vi "Labview Demo 2.vi"() -> ()   [LabVIEW 2016]
uses:
  C:/Program Files (x86)/Doodlebase/Transformer/Schemaport.Doodlebase.Transformer.dll
  Program Files (x86)/Doodlebase/Transformer/Schemaport.Doodlebase.Transformer.dll
panel:
  out "Network Success":bool
  in  "Variables":dbl
  in  "File Path Directory":path
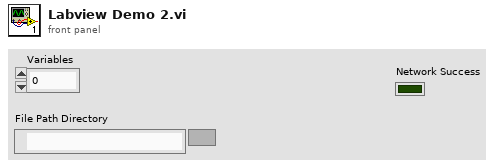
[diagram p1: front panel]
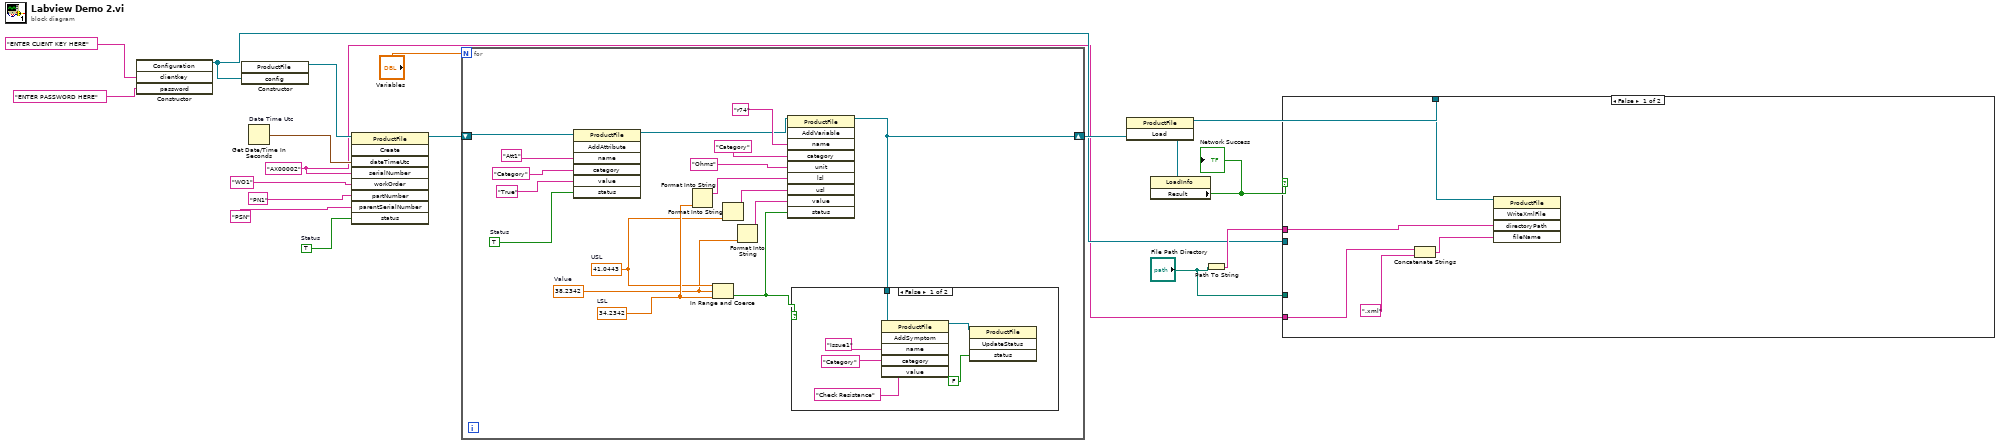
[diagram p0: block diagram]
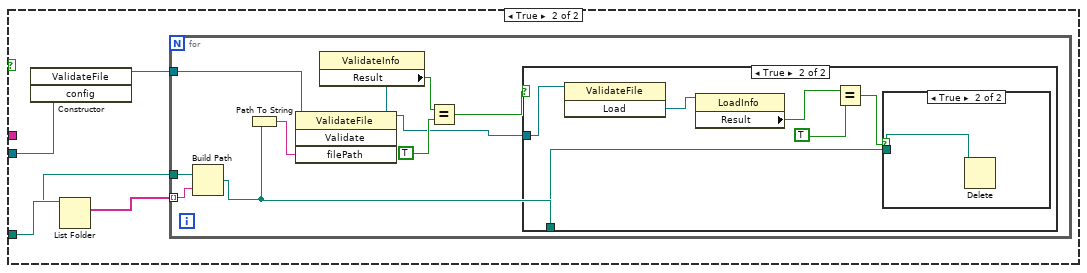
[diagram p2: hidden frame]
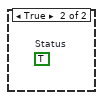
[diagram p5: hidden frame]
diagram:
  w12 = TRUE  # Status
  w1 = "AX00002"
  n1 = constructor class="Configuration"("clientkey"="ENTER CLIENT KEY HERE", "password"="ENTER PASSWORD HERE") -> (reference out=w3:refnum<k24>)  [unwired: 3 in, 4 out]
  n2 = constructor class="ProductFile"("config"=w3) -> (reference out=w16:refnum<k24>)  [unwired: 3 in, 3 out]
  n3 = Get Date/Time In Seconds "Date Time Utc"() -> (seconds since 1Jan1904=w11:timestamp)
  n4 = invoke class="ProductFile" method="Create"(reference=w16, "dateTimeUtc"=w11, "serialNumber"=w1, "workOrder"="WO1", "partNumber"="PN1", "parentSerialNumber"="PSN", "status"=w12) -> (reference out=w10:refnum<k24>)  [unwired: 2 in, 8 out]
  n5 = for {
    N: "Variables" -> [_]
    shift-right: [w19] -> w9
    shift-left: w10 -> [w35]
    w25 = 34.2342  # LSL
    w23 = 41.0443  # USL
    w20 = 38.2342  # Value
    w31 = TRUE  # Status
    n6 = invoke class="ProductFile" method="AddAttribute"(reference=w35, "name"="Att1", "category"="Category", "value"="True", "status"=w31) -> (reference out=w27:refnum<k24>)  [unwired: 2 in, 6 out]
    n7 = Format Into String(w25) -> (resulting string=w24:string)  [unwired: 3 in, 1 out]
    n8 = In Range and Coerce(upper limit=w23, x=w20, lower limit=w25) -> (In Range?=w26:bool)  [unwired: 1 out]
    n9 = Format Into String(w23) -> (resulting string=w22:string)  [unwired: 3 in, 1 out]
    n10 = Format Into String(w20) -> (resulting string=w21:string)  [unwired: 3 in, 1 out]
    n11 = invoke class="ProductFile" method="AddVariable"(reference=w27, "name"="r74", "category"="Category", "unit"="Ohms", "lsl"=w24, "usl"=w22, "value"=w21, "status"=w26) -> (reference out=w19:refnum<k24>)  [unwired: 2 in, 9 out]
    n12 = case shown="False" w26 {
      tunnel: w19 -> [w38 _]
      frame False {
        n13 = invoke class="ProductFile" method="AddSymptom"(reference=w38, "name"="Issue1", "category"="Category", "value"="Check Resistance") -> (reference out=w36:refnum<k24>)  [unwired: 2 in, 5 out]
        n14 = invoke class="ProductFile" method="UpdateStatus"(reference=w36, "status"=FALSE) -> ()  [unwired: 2 in, 4 out]
      }
      frame True {
        (unwired) TRUE  # Status
      }
    }
  }
  n15 = invoke class="ProductFile" method="Load"(reference=w9) -> (reference out=w5:refnum<k24>, "Load"=w6:refnum<k24>)  [unwired: 2 in, 1 out]
  n16 = property class="LoadInfo"(reference=w6) -> ("Result"=w8:bool)  [unwired: 1 in, 2 out]
  "Network Success" <- w8
  n17 = Path To String(path="File Path Directory") -> (string=w4:string)
  n18 = case shown="False" w8 {
    tunnel: w5 -> [w46 _]
    tunnel: w4 -> [w45 _]
    tunnel: w3 -> [_ w51]
    tunnel: "File Path Directory" -> [_ w49]
    tunnel: w1 -> [w43 _]
    frame False {
      n19 = Concatenate Strings(w43, ".xml") -> (w42:string)
      n20 = invoke class="ProductFile" method="WriteXmlFile"(reference=w46, "directoryPath"=w45, "fileName"=w42) -> ()  [unwired: 2 in, 5 out]
    }
    frame True {
      n21 = constructor class="ValidateFile"("config"=w51) -> (reference out=w50:refnum<k24>)  [unwired: 3 in, 3 out]
      n22 = List Folder(path=w49) -> (path out=w48:path, filenames=w47:string[])  [unwired: 3 in, 2 out]
      n23 = for {
        tunnel: w50 -> [w61]
        tunnel: w48 -> [w60]
        tunnel: w47 -> [w59] mode=indexing
        n24 = Build Path(base path=w60, name or relative path=w59) -> (appended path=w52:path)
        n25 = Path To String(path=w52) -> (string=w58:string)
        n26 = invoke class="ValidateFile" method="Validate"(reference=w61, "filePath"=w58) -> (reference out=w53:refnum<k24>, "Validate"=w57:refnum<k24>)  [unwired: 2 in, 2 out]
        n27 = property class="ValidateInfo"(reference=w57) -> ("Result"=w56:bool)  [unwired: 1 in, 2 out]
        n28 = Equal?(x=w56, y=TRUE) -> (x = y?=w54:bool)
        n29 = case shown="True" w54 {
          tunnel: w53 -> [_ w67]
          tunnel: w52 -> [_ w66]
          frame False {
          }
          frame True {
            n30 = invoke class="ValidateFile" method="Load"(reference=w67) -> ("Load"=w65:refnum<k24>)  [unwired: 2 in, 2 out]
            n31 = property class="LoadInfo"(reference=w65) -> ("Result"=w64:bool)  [unwired: 1 in, 2 out]
            n32 = Equal?(x=w64, y=TRUE) -> (x = y?=w62:bool)
            n33 = case shown="True" w62 {
              tunnel: w66 -> [_ w68]
              frame False {
              }
              frame True {
                n34 = Delete(path (use dialog)=w68) -> ()  [unwired: 4 in, 3 out]
              }
            }
          }
        }
      }
    }
  }
